vi "Clear-Receive.vi"(0 "DeviceType":T1=3 items=["PCI-CAN200"=7, "USB-CAN"=2, "USB-CAN200"=3], 1 "CANChannel":u32, 4 "DevInd":u32, 5 "错误输入":errorcluster) -> (7 "data":string, 11 "帧数据":string, 12 "每次接收完时间":u32, 13 "DeviceInd":u32, 14 "DeviceTypeOut":T1=3 items=["PCI-CAN200"=7, "USB-CAN"=2, "USB-CAN200"=3], 15 "Result":bool=TRUE, 17 "CANInd":u32, 18 "VCI_CAN_OBJ_R":T2={"ID"=96, 0, 0, 0, "TimeStamp"=0, "TimeFlag"=0, "SendType"=0, "RemoteFlag"=0, "ExternFlag"=0, "DataLen"=8, "Byte0"=0, "Byte1"=248, "Byte2"=17, "Byte3"=0, "Byte4"=0, "Byte5"=0, "Byte6"=0, "Byte7"=0, "Channel"=0, 77, 32} {"Byte7" format="%x"; "Byte6" format="%x"; "Byte5" format="%x"; "Byte4" format="%x"; "Byte3" format="%x"; "Byte2" format="%x"; "Byte1" format="%x"; "Byte0" format="%x"}, 19 "错误输出":errorcluster)   [LabVIEW 2013]
uses:
  DevType.ctl
  VCI_CAN.dll
panel:
  out "长度":string
  out "帧ID":string
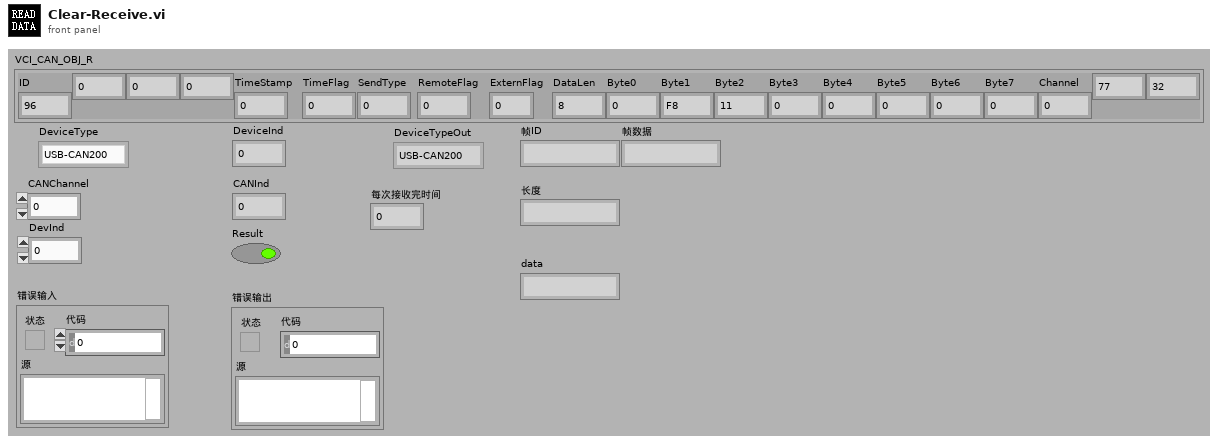
[diagram p1: front panel]
types:
  T1 = typedef "DevType.ctl" = u16
  T2 = cluster{"ID":u8, u8, u8, u8, "TimeStamp":u32, "TimeFlag":u8, "SendType":u8, "RemoteFlag":u8, "ExternFlag":u8, "DataLen":u8, "Byte0":u8, "Byte1":u8, "Byte2":u8, "Byte3":u8, "Byte4":u8, "Byte5":u8, "Byte6":u8, "Byte7":u8, "Channel":u8, u8, u8}
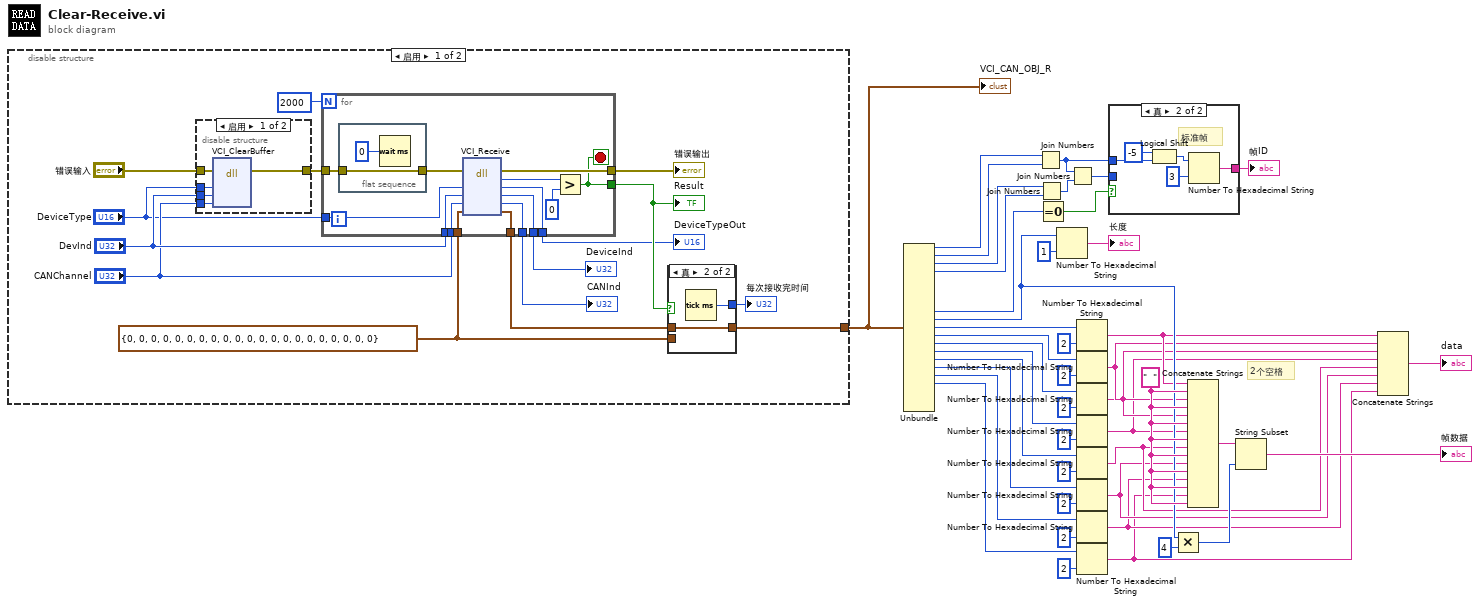
[diagram p0: block diagram]
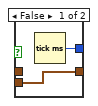
[diagram p3: hidden frame]
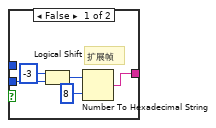
[diagram p5: hidden frame]
diagram:
  w23 = "  " ("字符串")
  # "2个空格"
  n1 = disable-structure shown="启用" {
    disable-tunnel: [w48 _] -> w10
    frame Enabled {
      w49 = T2 {"ID"=0, 0, 0, 0, "TimeStamp"=0, "TimeFlag"=0, "SendType"=0, "RemoteFlag"=0, "ExternFlag"=0, "DataLen"=0, "Byte0"=0, "Byte1"=0, "Byte2"=0, "Byte3"=0, "Byte4"=0, "Byte5"=0, "Byte6"=0, "Byte7"=0, "Channel"=0, 0, 0} ("VCI_CAN_OBJ_R 2")
      n2 = disable-structure shown="启用" {
        disable-tunnel: "错误输入" -> [w64 w65]
        disable-tunnel: "DevInd" -> [w63 _]
        disable-tunnel: [w62 w65] -> w56
        disable-tunnel: "CANChannel" -> [w61 _]
        disable-tunnel: "DeviceType" -> [w60 _]
        frame Enabled {
          n3 = dll-call lib="C:/Users/Administrator/Desktop/CAN/USBCAN/VCI_CAN.dll" fn="VCI_ClearBuffer"(error in=w64, "DeviceType"=w60, "DeviceInd"=w63, "CANInd"=w61) -> (error out=w62:errorcluster)  [unwired: 6 in, 1 out]
        }
        frame Disabled {
        }
      }
      n4 = for {
        N: 2000 -> [_]
        tunnel: [w78] -> w59
        tunnel: [w76] -> w47
        tunnel: "DeviceType" -> [w75]
        tunnel: "DevInd" -> [w74]
        tunnel: w56 -> [w73]
        tunnel: "CANChannel" -> [w71]
        tunnel: [w68] -> w54
        tunnel: [w70] -> w53
        tunnel: w49 -> [w69]
        tunnel: [w67] -> w46
        tunnel: [w66] -> w45
        stop <- w68 stop-if-true
        n5 = flat-sequence {
          tunnel: w73 -> [w80]
          tunnel: [w80] -> w72
          frame #0 {
            n6 = Wait (ms)(milliseconds to wait=u32 0 ("等待时间（毫秒）")) -> ()  [unwired: 1 out]
          }
        }
        n7 = dll-call lib="C:/Users/Administrator/Desktop/CAN/USBCAN/VCI_CAN.dll" fn="VCI_Receive"(error in=w72, "DeviceType"=w75, "DeviceInd"=w74, "CANInd"=w71, "VCI_CAN_OBJ_R"=w69) -> (error out=w78:errorcluster, "返回类型"=w77:u32, "DeviceType"=w76:u32, "DeviceInd"=w67:u32, "CANInd"=w66:u32, "VCI_CAN_OBJ_R"=w70:T2)  [unwired: 2 in, 1 out]
        n8 = Greater?(x=w77, y=u32 0) -> (0:w68:bool)
      }
      "错误输出" <- w59
      "Result" <- w54
      "DeviceTypeOut" <- w47
      "DeviceInd" <- w46
      "CANInd" <- w45
      n9 = case shown="真" w54 {
        tunnel: w53 -> [_ w84]
        tunnel: [w83 w85] -> w52
        tunnel: [w82 w84] -> w48
        tunnel: w49 -> [w82 _]
        frame False {
          n10 = Tick Count (ms)() -> (millisecond timer value=w83:u32)
        }
        frame True {
          n11 = Tick Count (ms)() -> (millisecond timer value=w85:u32)
        }
      }
      "每次接收完时间" <- w52
    }
    frame Disabled {
    }
  }
  "VCI_CAN_OBJ_R" <- w10
  n12 = Unbundle(w10) -> ("ID"=w43:u8, w44:u8, w42:u8, w41:u8, "ExternFlag"=w18:u8, "DataLen"=w22:u8, "Byte0"=w40:u8, "Byte1"=w39:u8, "Byte2"=w37:u8, "Byte3"=w36:u8, "Byte4"=w35:u8, "Byte5"=w34:u8, "Byte6"=w33:u8, "Byte7"=w32:u8)  [unwired: 7 out]
  n13 = Join Numbers(hi=w43, lo=w44) -> ((hi.lo)=w14:u16)
  n14 = Join Numbers(hi=w42, lo=w41) -> ((hi.lo)=w15:u16)
  n15 = Equal To 0?(x=w18) -> (x = 0?=w17:bool)
  n16 = Number To Hexadecimal String(1:i16 1 ("宽度(-)"), 2:w22) -> (0:→"长度":string)
  n17 = Join Numbers(hi=w14, lo=w15) -> ((hi.lo)=w16:u32)
  n18 = Number To Hexadecimal String(1:i16 2 ("宽度(-)"), 2:w40) -> (0:w9:string)
  n19 = Number To Hexadecimal String(1:i16 2 ("宽度(-)"), 2:w39) -> (0:w8:string)
  n20 = Number To Hexadecimal String(1:i16 2 ("宽度(-)"), 2:w37) -> (0:w7:string)
  n21 = Number To Hexadecimal String(1:i16 2 ("宽度(-)"), 2:w36) -> (0:w6:string)
  n22 = Number To Hexadecimal String(1:i16 2 ("宽度(-)"), 2:w35) -> (0:w5:string)
  n23 = Number To Hexadecimal String(1:i16 2 ("宽度(-)"), 2:w34) -> (0:w4:string)
  n24 = Number To Hexadecimal String(1:i16 2 ("宽度(-)"), 2:w33) -> (0:w3:string)
  n25 = Number To Hexadecimal String(1:i16 2 ("宽度(-)"), 2:w32) -> (0:w2:string)
  n26 = case shown="真" w17 {
    tunnel: [w89 w92] -> w13
    tunnel: w16 -> [w87 _]
    tunnel: w14 -> [_ w91]
    frame False {
      # "扩展帧"
      n27 = Logical Shift(y=i8 -3, x=w87) -> (x << y=w88:u32)
      n28 = Number To Hexadecimal String(1:i16 8 ("宽度(-)"), 2:w88) -> (0:w89:string)
    }
    frame True {
      # "标准帧"
      n29 = Logical Shift(y=i8 -5, x=w91) -> (x << y=w94:u16)
      n30 = Number To Hexadecimal String(1:i16 3 ("宽度(-)"), 2:w94) -> (0:w92:string)
    }
  }
  "帧ID" <- w13
  n31 = Multiply(x=w22, y=u8 4) -> (x*y=w20:u8)
  n32 = Concatenate Strings(w9, w23, w8, w23, w7, w23, w6, w23, w5, w23, w4, w23, w3, w23, w2, w23) -> (w19:string)
  n33 = String Subset(string=w19, length (rest)=w20) -> (substring=→"帧数据":string)  [unwired: 1 in]
  n34 = Concatenate Strings(w9, w8, w7, w6, w5, w4, w3, w2) -> (→"data":string)
